vi "Flight Gear Interface Main Page.vi"(8 "error in (no error)":errorcluster, 11 "Node Ptr":T1 format="%.0x") -> (0 "error out":errorcluster)   [LabVIEW 2010, in "Flight Gear Interface Custom Device.lvlib"]
uses:
  Flight Gear Interface Custom Device.lvlib
  <vilib>/NI VeriStand/Custom Device API/Custom Device Item Ref.ctl
  <vilib>/NI VeriStand/Custom Device API/Get Item Property (I32).vi
  <vilib>/NI VeriStand/Custom Device API/Get Item Property (String).vi
  <vilib>/NI VeriStand/Custom Device API/Get Item Property (U16).vi
  <vilib>/NI VeriStand/Custom Device API/Set Item Property (I32).vi
  <vilib>/NI VeriStand/Custom Device API/Set Item Property (String).vi
  <vilib>/NI VeriStand/Custom Device API/Set Item Property (U16).vi
  <vilib>/NI Veristand/Custom Device API/Custom Device API.lvlib
panel:
  in  "Port":u16
  in  "Set To Current":bool
  in  "Flight Gear Target IP Address":string
  in  "Rate Decimation":i32
  in  "Processor Assignment":i32
  in  "Header":cluster{"Section Name":string}={"Section Name"="Flight Gear Interface Settings"}
  in  "Description":string
  in  "Name":string
  in  "Delete":bool
  # "(-2 is Auto)"
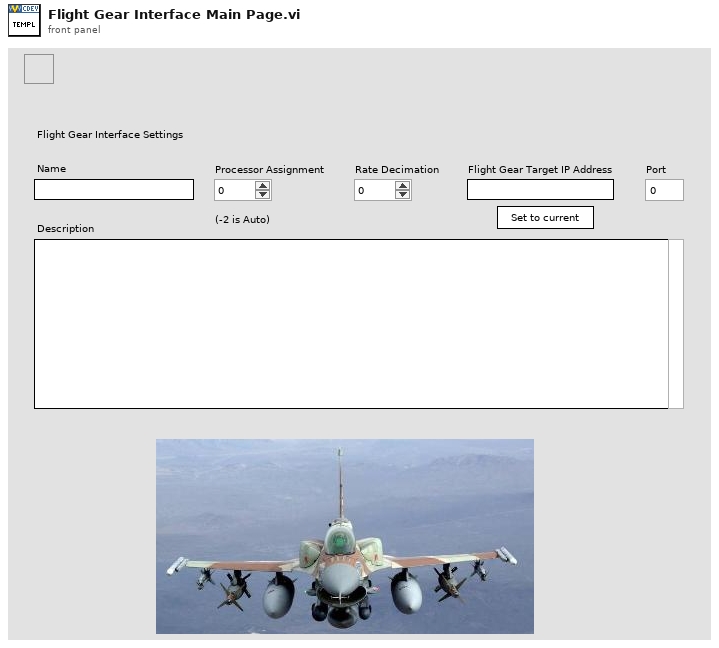
[diagram p1: front panel]
types:
  T1 = typedef "Custom Device API.lvlib/Custom Device Item Ref.ctl" = u64
  T2 = typedef "Custom Device API.lvlib/Custom Device Item Info.ctl" = cluster{"Name":string, "Is Channel":bool, "GUID":string}
  T3 = typedef "Custom Device API.lvlib/Custom Device Commands.ctl" = enum16{"Default", "Item renamed", "Shutdown", "Dynamic button pressed"}
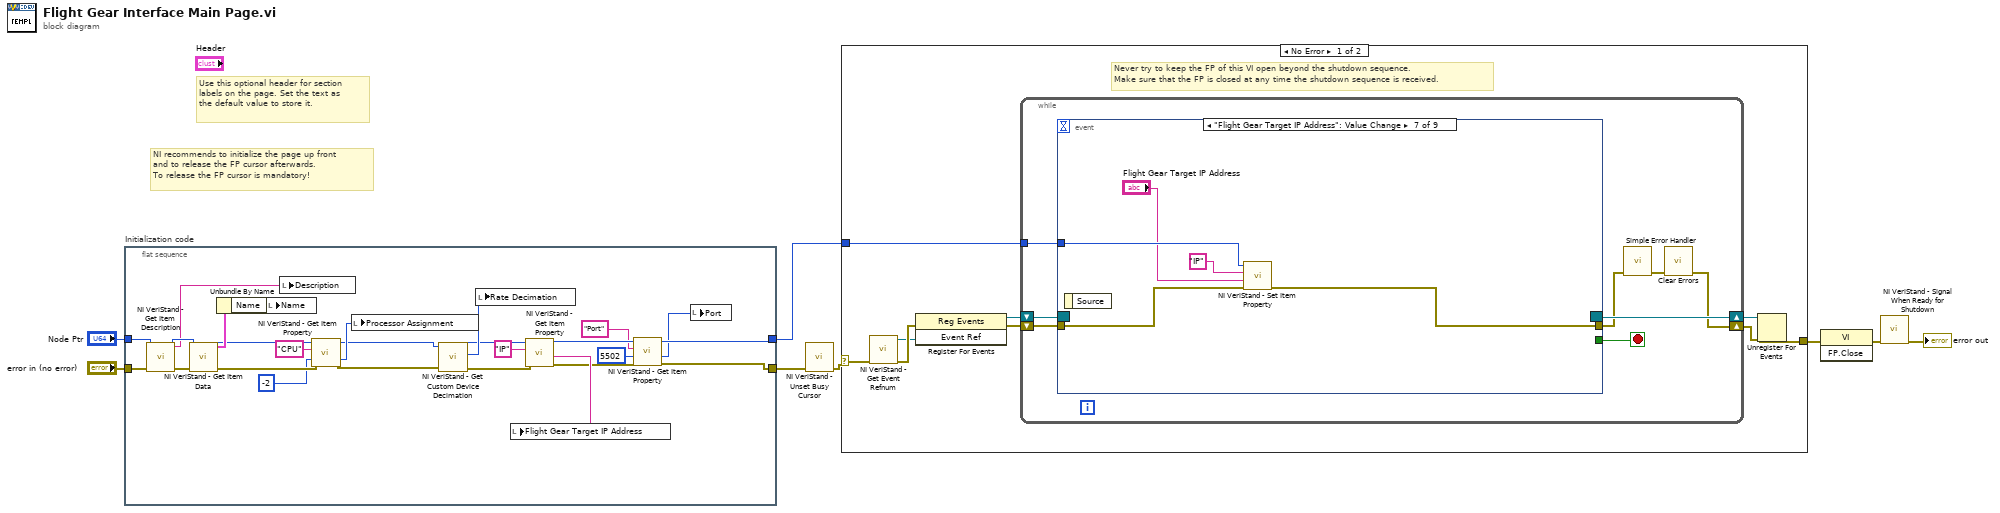
[diagram p0: block diagram]
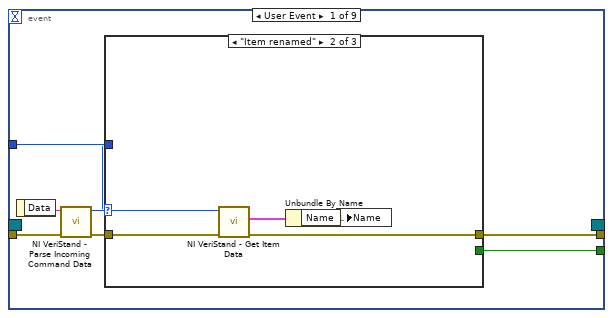
[diagram p2: hidden frame]
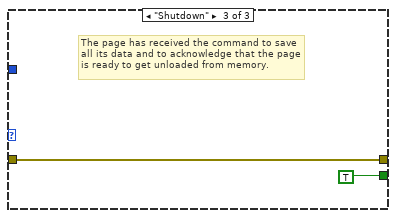
[diagram p4: hidden frame]
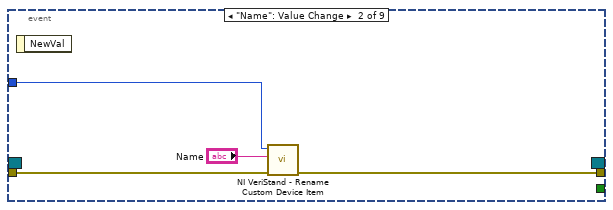
[diagram p5: hidden frame]
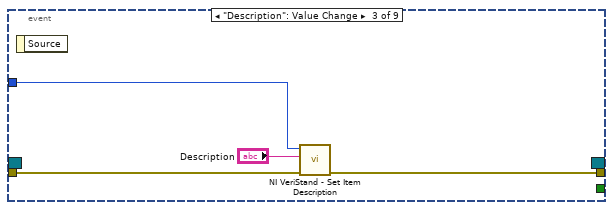
[diagram p6: hidden frame]
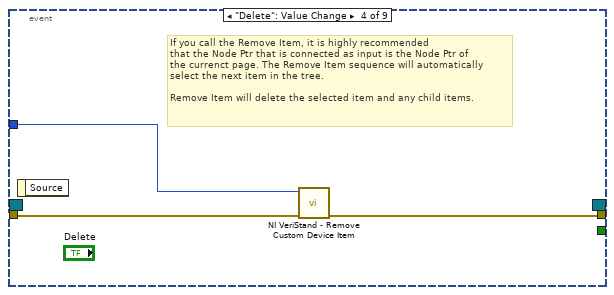
[diagram p7: hidden frame]
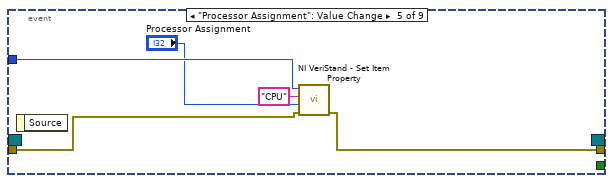
[diagram p8: hidden frame]
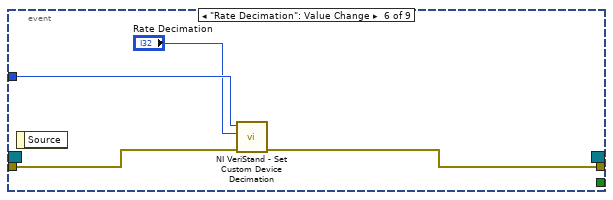
[diagram p9: hidden frame]
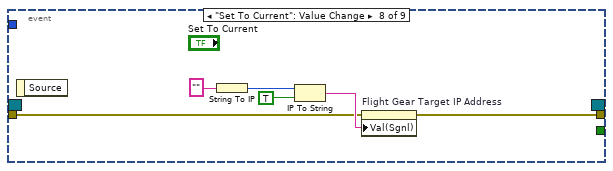
[diagram p10: hidden frame]
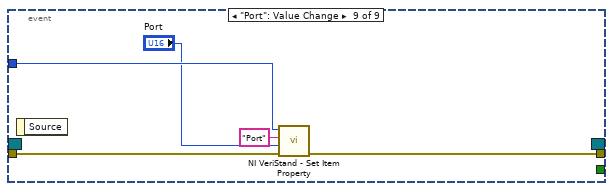
[diagram p11: hidden frame]
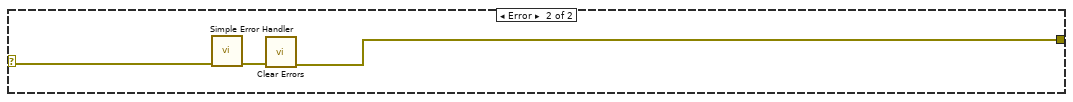
[diagram p12: hidden frame]
diagram:
  # "Use this optional header for section labels on the page. Set the text as the default value to store it."
  # "NI recommends to initialize the page up front\nand to release the FP cursor afterwards.\nTo release the FP cursor is mandatory!"
  n1 = flat-sequence "Initialization code" {
    tunnel: "error in (no error)" -> [w33]
    tunnel: "Node Ptr" -> [w32]
    tunnel: [w12] -> w4
    tunnel: [w13] -> w1
    frame #0 {
      n2 = call <vilib>:"NI VeriStand - Get Item Description.vi"("error in (no error)"=w33, "Item Ref in"=w32) -> ("error out"=w30:errorcluster, "Description"=w31:string, "Item Ref out"=w34:T1)  [unwired: 7 out]
      n3 = call <vilib>:"NI VeriStand - Get Item Data.vi"("error in (no error)"=w30, "Item Ref in"=w34) -> ("error out"=w27:errorcluster, "Item Info"=w29:T2, "Item Ref out"=w26:T1)  [unwired: 7 out]
      n4 = Unbundle By Name(w29) -> ("Name"=w28:string)
      n5 = local write "Name"(w28) -> ()
      n6 = local write "Description"(w31) -> ()
      n7 = call-poly <vilib>:"NI VeriStand - Get Item Property.vi"("error in (no error)"=w27, "Default Value"=-2, "Property Name"="CPU", "Item Ref in"=w26) -> ("error out"=w22:errorcluster, "Value"=w23:i32, "Item Ref out"=w21:T1)  [unwired: 4 in, 1 out]
      n8 = local write "Processor Assignment"(w23) -> ()
      n9 = call <vilib>:"NI VeriStand - Get Custom Device Decimation.vi"("error in (no error)"=w22, "Device Ref in"=w21) -> ("error out"=w19:errorcluster, "Decimation"=w20:i32, "Device Ref out"=w18:T1)  [unwired: 7 in]
      n10 = local write "Rate Decimation"(w20) -> ()
      n11 = call-poly <vilib>:"NI VeriStand - Get Item Property.vi"("error in (no error)"=w19, "Property Name"="IP", "Item Ref in"=w18) -> ("error out"=w15:errorcluster, "Value"=w16:string, "Item Ref out"=w14:T1)  [unwired: 5 in, 1 out]
      n12 = local write "Flight Gear Target IP Address"(w16) -> ()
      n13 = call-poly <vilib>:"NI VeriStand - Get Item Property.vi"("error in (no error)"=w15, "Default Value"=u16 5502, "Property Name"="Port", "Item Ref in"=w14) -> ("error out"=w12:errorcluster, "Value"=w9:u16, "Item Ref out"=w13:T1)  [unwired: 4 in, 1 out]
      n14 = local write "Port"(w9) -> ()
    }
  }
  n15 = call <vilib>:"NI VeriStand - Unset Busy Cursor.vi"("error in (no error)"=w4) -> ("error out"=w3:errorcluster)  [unwired: 10 out]
  n16 = case shown="No Error" w3 {
    selector: w3 -> [w35 w105]
    tunnel: [w40 w103] -> w8
    tunnel: w1 -> [w36 _]
    frame No Error {
      # "Never try to keep the FP of this VI open beyond the shutdown sequence.\nMake sure that the FP is closed at any time the shutdown sequence is received."
      n17 = call <vilib>:"NI VeriStand - Get Event Refnum.vi"("error in (no error)"=w35) -> ("error out"=w43:errorcluster, "Event Ref"=w39:refnum<user-event>)  [unwired: 9 out]
      n18 = register-events(error in=w43, w39) -> (reference out=w37:refnum<event-registration>, error out=w38:errorcluster)  [unwired: 1 in]
      n19 = while {
        tunnel: w36 -> [w47]
        shift-right: [w44] -> w41
        shift-left: w38 -> [w50]
        shift-right: [w51] -> w42
        shift-left: w37 -> [w49]
        stop <- w48 stop-if-true
        n20 = event shown="[6] \"Flight Gear Target IP Address\": Value Change" {
          selector: w49 -> [_ _ _ _ _ _ _ _ _]
          dyn-events: [_ _ _ _ _ _ _ _ _] -> w51
          timeout: _ -> [_ _ _ _ _ _ _ _ _]
          tunnel: w50 -> [w58 w70 w73 w77 w82 w86 w91 w93 w101]
          tunnel: [w54 _ _ _ _ _ _ _ _] -> w48
          tunnel: [w53 w69 w72 w76 w78 w84 w87 w92 w100] -> w46
          tunnel: w47 -> [w52 w68 w74 w75 w81 w85 w90 _ w102]
          event User Event {
            n21 = event-data() -> ("Data"=w57:string)  [unwired: 1 out]
            n22 = call <vilib>:"NI VeriStand - Parse Incoming Command Data.vi"("error in (no error)"=w58, "Data"=w57) -> ("error out"=w56:errorcluster, "Action"=w55:T3)  [unwired: 8 out]
            n23 = case shown="\"Item renamed\"" w55 {
              tunnel: w56 -> [w59 w64 w65]
              tunnel: [_ _ TRUE] -> w54
              tunnel: [w59 w61 w65] -> w53
              tunnel: w52 -> [_ w63 _]
              frame "Default", Default {
              }
              frame "Item renamed" {
                n24 = call <vilib>:"NI VeriStand - Get Item Data.vi"("error in (no error)"=w64, "Item Ref in"=w63) -> ("error out"=w61:errorcluster, "Item Info"=w62:T2)  [unwired: 8 out]
                n25 = Unbundle By Name(w62) -> ("Name"=w60:string)
                n26 = local write "Name"(w60) -> ()
              }
              frame "Shutdown" {
                # "The page has received the command to save all its data and to acknowledge that the page is ready to get unloaded from memory."
              }
            }
          }
          event "Name": Value Change {
            n27 = event-data() -> ()  [unwired: 2 out]
            n28 = call <vilib>:"NI VeriStand - Rename Custom Device Item.vi"("error in (no error)"=w70, "New Name"="Name", "Item Ref in"=w68) -> ("error out"=w69:errorcluster)  [unwired: 8 out]
          }
          event "Description": Value Change {
            n29 = event-data() -> ()  [unwired: 2 out]
            n30 = call <vilib>:"NI VeriStand - Set Item Description.vi"("error in (no error)"=w73, "Description"="Description", "Item Ref in"=w74) -> ("error out"=w72:errorcluster)  [unwired: 8 out]
          }
          event "Delete": Value Change {
            # "If you call the Remove Item, it is highly recommended\nthat the Node Ptr that is connected as input is the Node Ptr of\nthe currenct page. The Remove Item sequence will automatically\nselect the next item in the tree.\n\nRemove Item will delete the selected item and any child items."
            n31 = event-data() -> ()  [unwired: 2 out]
            n32 = call <vilib>:"NI VeriStand - Remove Custom Device Item.vi"("error in (no error)"=w77, "Item Ref in"=w75) -> ("error out"=w76:errorcluster)  [unwired: 1 in, 8 out]
          }
          event "Processor Assignment": Value Change {
            n33 = event-data() -> ()  [unwired: 2 out]
            n34 = call-poly <vilib>:"NI VeriStand - Set Item Property.vi"("error in (no error)"=w82, "Value"="Processor Assignment", "Property Name"="CPU", "Item Ref in"=w81) -> ("error out"=w78:errorcluster)  [unwired: 5 in, 2 out]
          }
          event "Rate Decimation": Value Change {
            n35 = event-data() -> ()  [unwired: 2 out]
            n36 = call <vilib>:"NI VeriStand - Set Custom Device Decimation.vi"("error in (no error)"=w86, "Decimation"="Rate Decimation", "Device Ref in"=w85) -> ("error out"=w84:errorcluster)  [unwired: 7 in, 1 out]
          }
          event "Flight Gear Target IP Address": Value Change {
            n37 = event-data() -> ()  [unwired: 2 out]
            n38 = call-poly <vilib>:"NI VeriStand - Set Item Property.vi"("error in (no error)"=w91, "Value"="Flight Gear Target IP Address", "Property Name"="IP", "Item Ref in"=w90) -> ("error out"=w87:errorcluster)  [unwired: 5 in, 2 out]
          }
          event "Set To Current": Value Change {
            n39 = event-data() -> ()  [unwired: 2 out]
            n40 = String To IP(1:"" ("name")) -> (0:w96:u32)
            n41 = IP To String(1:TRUE ("dot notation? (F)"), 2:w96) -> (0:w94:string)
            n42 = property on="Flight Gear Target IP Address" class="Str"(error in=w93, "Val(Sgnl)"=w94) -> (error out=w92:errorcluster)  [unwired: 1 in, 1 out]
          }
          event "Port": Value Change {
            n43 = event-data() -> ()  [unwired: 2 out]
            n44 = call-poly <vilib>:"NI VeriStand - Set Item Property.vi"("error in (no error)"=w101, "Value"="Port", "Property Name"="Port", "Item Ref in"=w102) -> ("error out"=w100:errorcluster)  [unwired: 5 in, 2 out]
          }
        }
        n45 = call <vilib>:"Simple Error Handler.vi"("error in (no error)"=w46) -> ("error out"=w45:errorcluster)  [unwired: 1 in, 7 out]
        n46 = call <vilib>:"Clear Errors.vi"("error in (no error)"=w45) -> ("error out"=w44:errorcluster)  [unwired: 6 out]
      }
      n47 = Unregister For Events(event registration refnum=w42, error in=w41) -> (error out=w40:errorcluster)
    }
    frame Error {
      n48 = call <vilib>:"Simple Error Handler.vi"("error in (no error)"=w105) -> ("error out"=w104:errorcluster)  [unwired: 1 in, 7 out]
      n49 = call <vilib>:"Clear Errors.vi"("error in (no error)"=w104) -> ("error out"=w103:errorcluster)  [unwired: 6 out]
    }
  }
  n50 = invoke class="VI" method="FP.Close"(error in=w8) -> (error out=w7:errorcluster)  [unwired: 2 in, 2 out]
  n51 = call <vilib>:"NI VeriStand - Signal When Ready for Shutdown.vi"("error in (no error)"=w7) -> ("error out"=→"error out":errorcluster)  [unwired: 10 out]
